vi "SetObjectConfiguration.vi"(8 "error in (no error)":errorcluster, 9 "Values":variant[](array[variant]), 10 "Keys":string[](array[string]), 11 "SMO":refnum<class "SMO.lvclass">) -> (0 "error out":errorcluster, 2 "keys dup":string[](array[string]), 3 "SMO out":refnum<class "SMO.lvclass">)   [LabVIEW 2013, in "SMO.lvclass"]
uses:
  SMO.lvclass
  Support/Attribute.Config/Attribute.Config.lvclass/Attribute.Config.ctl
  <vilib>/LabVIEW Open Source Project/Configuration Manager/Manager/ConfigManager.lvclass
  Support/Attribute.Config/Attribute.Config.lvclass
panel:
  # "For instructions on how to use the JKI State Machine Objects, examples and video tutorials, visit:\nhttp://jki.net/state-machine-objects/\n\nJKI State Machine Objects™\nhttp://jki.net/state-machine-objects/\nCopyright (C) 2005-2015, JKI <info@jki.net>\nALL RIGHTS RESERVED"
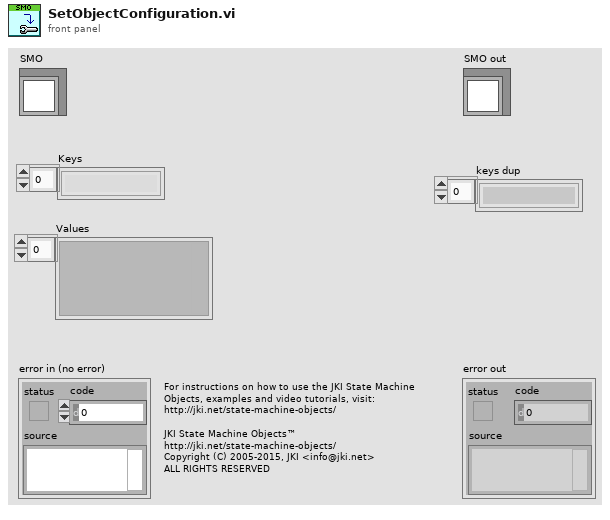
[diagram p1: front panel]
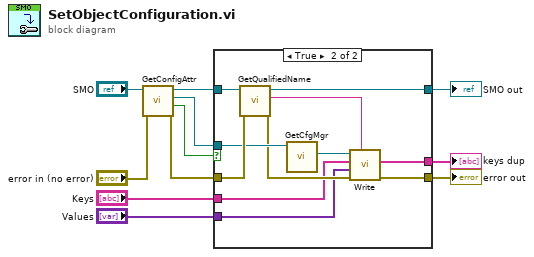
[diagram p0: block diagram]
diagram:
  n1 = call "GetConfigAttr.vi"("error in (no error)"="error in (no error)", "SMO in"="SMO") -> ("error out"=w4:errorcluster, "found"=w7:bool, "Attribute.Config"=w6:refnum<class "Attribute.Config.lvclass">, "SMO out"=w8:refnum<class "SMO.lvclass">)  [unwired: 6 in]
  n2 = case shown="True" w7 {
    tunnel: w6 -> [_ w22]
    tunnel: w8 -> [w14 w25]
    tunnel: [w14 w24] -> w11
    tunnel: w4 -> [w13 w23]
    tunnel: [w13 w18] -> w10
    tunnel: "Keys" -> [w12 w17]
    tunnel: "Values" -> [_ w16]
    tunnel: [w12 w15] -> w1
    frame False {
    }
    frame True {
      n3 = call "GetQualifiedName.vi"("error in (no error)"=w23, "SMO"=w25) -> ("error out"=w19:errorcluster, "Qualified Name"=w21:string, "SMO out"=w24:refnum<class "SMO.lvclass">)  [unwired: 7 in]
      n4 = call "GetCfgMgr.vi"("Attribute.Config in"=w22) -> ("CfgMgr"=w20:refnum<class "ConfigManager.lvclass">)  [unwired: 9 in, 1 out]
      n5 = call <vilib>:"Write.vi"("Qualified Name"=w21, "error in (no error)"=w19, "Values"=w16, "keys"=w17, "ConfigManager in"=w20) -> ("error out"=w18:errorcluster, "keys dup"=w15:string[])  [unwired: 4 in, 1 out]
    }
  }
  "error out" <- w10
  "SMO out" <- w11
  "keys dup" <- w1
